vi "DC Voltage Source (DAQmx).vi"() -> ()   [LabVIEW 2013]
uses:
  <vilib>/DAQmx/write.llb/DAQmx Write (Analog DBL 1Chan 1Samp).vi
  <vilib>/DAQmx/create/channels.llb/DAQmx Create Channel (AO-Voltage-Basic).vi
  <vilib>/DAQmx/miscellaneous.llb/DAQmx Fill In Error Info.vi
panel:
  in  "Knob":dbl(knob) min=-10.0 max=10.0 step=0.1 scale=-4.0..4.0 scale format="%#.4g"
  in  "physical channels":tag
  in  "stop":bool
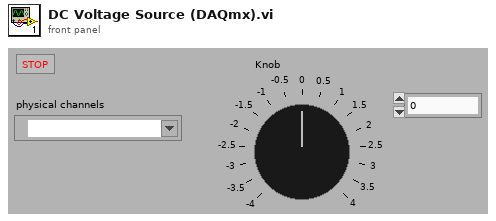
[diagram p1: front panel]
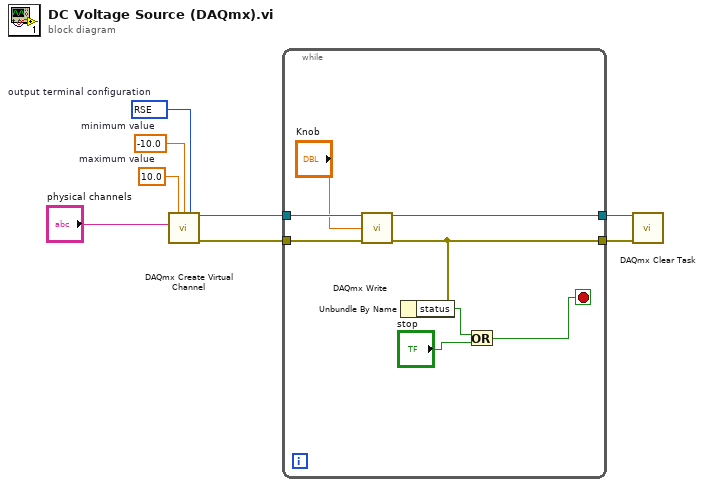
[diagram p0: block diagram]
diagram:
  w6 = 10083 items=["default"=-1, "RSE"=10083, "NRSE"=10078, "Differential"=10106, "Pseudodifferential"=12529]  # output terminal configuration
  w7 = -10.0  # minimum value
  w8 = 10.0  # maximum value
  n1 = call-poly <vilib>:"DAQmx Create Virtual Channel.vi"("maximum value"=w8, "minimum value"=w7, "output terminal configuration"=w6, "physical channels"="physical channels") -> ("task out"=w5:refnum<k21>, "error out"=w4:errorcluster)  [unwired: 5 in, 5 out]
  n2 = while {
    tunnel: w5 -> [w16]
    tunnel: w4 -> [w15]
    tunnel: [w14] -> w3
    tunnel: [w13] -> w2
    stop <- w9 stop-if-true
    n3 = call-poly <vilib>:"DAQmx Write.vi"("task/channels in"=w16, "data"="Knob", "error in"=w15) -> ("task out"=w13:refnum<k21>, "error out"=w14:errorcluster)  [unwired: 1 in, 10 out]
    n4 = Unbundle By Name(w14) -> ("status"=w11:bool)
    n5 = Or(x=w11, y="stop") -> (x .or. y?=w9:bool)
  }
  n6 = call <vilib>:"DAQmx Clear Task.vi"("task in"=w2, "error in"=w3) -> ()  [unwired: 14 out]
